vi "sig.delegate_pausing_lua.vi"(5 "LuaVIEW reference":T1) -> (15 "error out":errorcluster)   [LabVIEW 2012]
doc: "Redelegate the built-in handling of pause and resume signals. When a task starts, the handling is already delegated to the built-in mechanism. This function is therefore only useful when your task performs custom handling of pause/resume signals for a limited time.\nErrors:\nFunction must be called from a task context but was not."
uses:
  typedefs/t_LuaVIEW Reference.ctl
  typedefs/t_LuaVIEW Task Signals.ctl
  typedefs/t_LuaVIEW Task State Methods.ctl
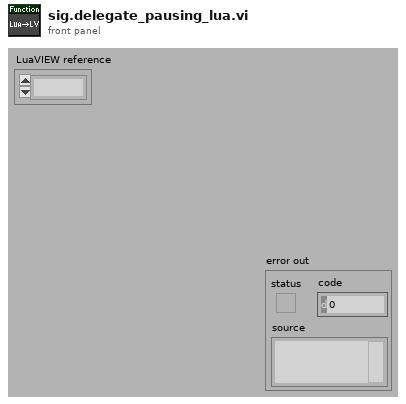
[diagram p1: front panel]
types:
  T1 = typedef "t_LuaVIEW Reference.ctl" = refnum<k1>
  T2 = typedef "t_LuaVIEW Task State Methods.ctl" = enum16{"cleanup", "set initial", "set mode", "set active mode", "set error", "get task info", "get script info", "set signal", "clear signal", "test handled", "test delegated", "test signal", "handle signal", "delegate signal", "allow signal", "disallow signal", "disallow all", "signals?", "delegated signals?", "protection++", "protection--", "protection=0", "message", "next message", "pop message", "message available?", "force stop", "set swap preps", "apply swap preps"}
  T3 = typedef "t_LuaVIEW Task Signals.ctl" = enum32{"resume", "pause", "swap", "stop", "confirm"}
  T4 = typedef "t_LuaVIEW Task State Pane.ctl" = refnum<vi>
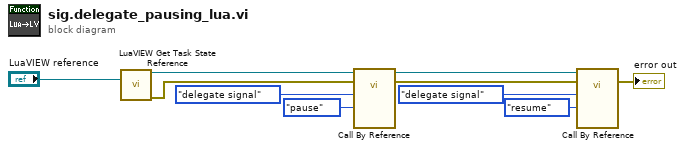
[diagram p0: block diagram]
diagram:
  n1 = call "LuaVIEW Get Task State Reference.vi"("LuaVIEW reference in"="LuaVIEW reference") -> ("task state reference"=w10:T4, "error out"=w6:errorcluster)  [unwired: 12 in, 1 out]
  n2 = call-by-ref "?"(reference=w10, error in=w6, "method"=t_LuaVIEW_Task_State_Methods."delegate signal", "signal"=t_LuaVIEW_Task_Signals."pause") -> (reference out=w1:T4, error out=w2:errorcluster)  [unwired: 9 in, 5 out]
  n3 = call-by-ref "?"(reference=w1, error in=w2, "method"=t_LuaVIEW_Task_State_Methods."delegate signal", "signal"=t_LuaVIEW_Task_Signals."resume") -> (error out=→"error out":errorcluster)  [unwired: 9 in, 6 out]
